vi "Convert-TIFF-to-FITS-3dU16.vi"(0 "file path":path) -> ()   [LabVIEW 2011]
panel:
  out "TIFF-strings":string[](array[string])
  out "FITS":T1={"BITPIX"=16.0, "NAXIS"=3.0, "NAXIS1"=300.0, "NAXIS2"=300.0, "NAXIS3"=1.0, "BZERO"=0.0, "BSCALE"=1.0}
  out "error out":errorcluster
  # "ASIFITSVIew OK\nIJ OK"
  # "SIMPLE   =  T\n...\nEND"
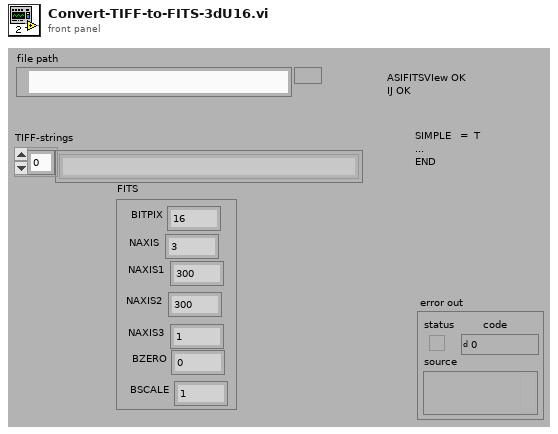
[diagram p1: front panel]
types:
  T1 = cluster{"BITPIX":sgl, "NAXIS":sgl, "NAXIS1":sgl, "NAXIS2":sgl, "NAXIS3":sgl, "BZERO":sgl, "BSCALE":sgl}
  T2 = cluster{"Tiff refnum":refnum<file>, "Byte-Reihenfolge (0:Big-Endian, 2:LSB)":enum16{"big-endian, network order", "native, host order", "little-endian"}}
  T3 = enum16{"big-endian, network order", "native, host order", "little-endian"}
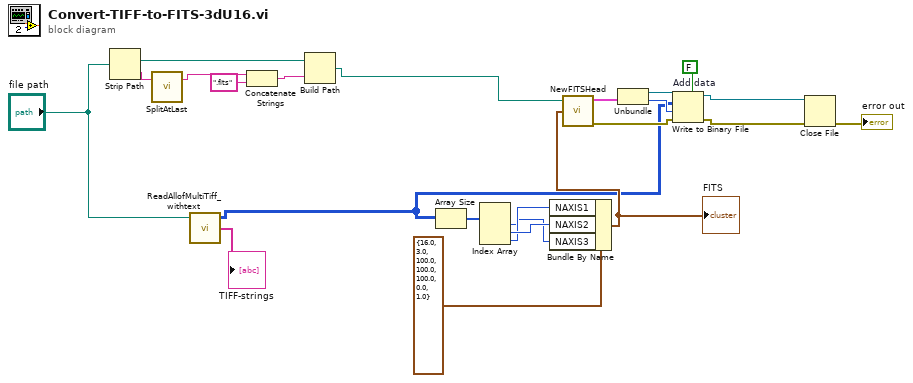
[diagram p0: block diagram]
diagram:
  n1 = Strip Path(path="file path") -> (stripped path=w19:path, name=w23:string)
  n2 = call "SplitAtLast.vi"("In-String"=w23) -> ("Front (default)"=w22:string)  [unwired: 1 in, 1 out]
  n3 = call "ReadAllofMultiTiff_withtext.vi"("file path"="file path") -> ("strings"=→"TIFF-strings":string[], "16-bit pixmaps"=w2:i16[][][])  [unwired: 2 in, 1 out]
  n4 = Concatenate Strings(w22, ".fits" ("String")) -> (w20:string)
  n5 = Build Path(base path=w19, name or relative path=w20) -> (appended path=w5:path)
  n6 = Array Size(array=w2) -> (size(s)=w17:i32[])
  n7 = Index Array(array=w17) -> (element #1=w7:i32, element #2=w16:i32, element #3=w8:i32)  [unwired: 3 in]
  n8 = Bundle By Name(cluster=T1 {"BITPIX"=16.0, "NAXIS"=3.0, "NAXIS1"=100.0, "NAXIS2"=100.0, "NAXIS3"=100.0, "BZERO"=0.0, "BSCALE"=1.0} ("FITS"), "NAXIS1"=w8, "NAXIS2"=w16, "NAXIS3"=w7) -> (w9:T1)
  "FITS" <- w9
  n9 = call "NewFITSHead.vi"("file path"=w5, "FITS"=w9) -> ("FITS file"=w15:T2, "error out"=w12:errorcluster)  [unwired: 2 in, 1 out]
  n10 = Unbundle(w15) -> ("Tiff refnum"=w14:refnum<file>, "Byte-Reihenfolge (0:Big-Endian, 2:LSB)"=w13:T3)
  n11 = Write to Binary File "Add data"(file (use dialog)=w14, data=w2, error in=w12, 5:FALSE ("prepend array or string size? (T)"), 9:w13) -> (refnum out=w10:refnum<file>, error out=w11:errorcluster)  [unwired: 2 out]
  n12 = Close File(refnum=w10, error in=w11) -> (error out=→"error out":errorcluster)  [unwired: 1 out]
